vi "test Verify with Multi Scrubber.vi"(8 "error in":errorcluster, 11 "Test Case In":refnum<class "LUnit Extensions Tests.lvclass">) -> (0 "error out":errorcluster, 3 "Test Case Out":refnum<class "LUnit Extensions Tests.lvclass">)   [LabVIEW 2020, in "LUnit Extensions Tests.lvclass"]
uses:
  LUnit Extensions Tests.lvclass
  LUnit Extensions Tests.lvclass/LUnit Extensions Tests.ctl
  240f995d-3744-484a-8956-6f48e6079b93.vi
  Source/Approval Tests/Regex Scrubber/Regex Scrubber.lvclass
  Source/Approval Tests/Options/Options.lvclass
  C:/Users/SAS/Desktop/ApprovalTests.LabVIEW/Source/Approval Tests/Regex Scrubber/Regex Scrubber.lvclass
  C:/Users/SAS/Desktop/ApprovalTests.LabVIEW/Source/Approval Tests/Scrubber/Scrubber.lvclass
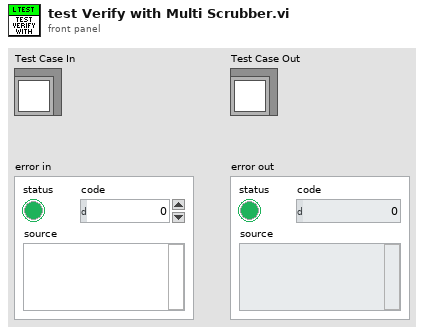
[diagram p1: front panel]
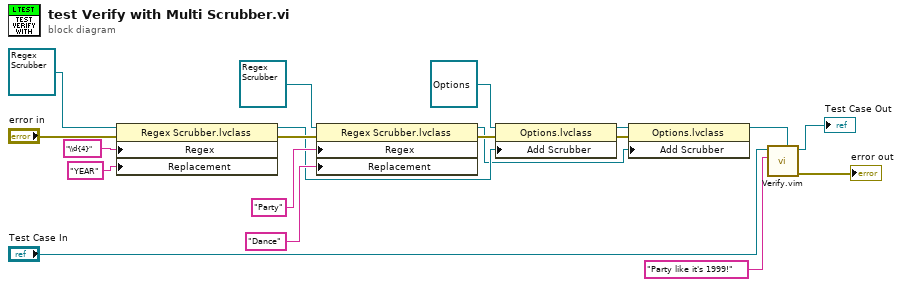
[diagram p0: block diagram]
diagram:
  n1 = property class="Regex Scrubber.lvclass"(reference=refnum<class "Regex Scrubber.lvclass"> refnum ("Approval Tests.lvlib:Regex Scrubber.lvclass"), error in="error in", "Regex"="\\d{4}", "Replacement"="YEAR") -> (reference out=w5:refnum<class "Regex Scrubber.lvclass">, error out=w18:errorcluster)
  n2 = property class="Regex Scrubber.lvclass"(reference=refnum<class "Regex Scrubber.lvclass"> refnum ("Approval Tests.lvlib:Regex Scrubber.lvclass"), error in=w18, "Regex"="Party", "Replacement"="Dance") -> (reference out=w2:refnum<class "Regex Scrubber.lvclass">, error out=w6:errorcluster)
  n3 = property class="Options.lvclass"(reference=refnum<class "Options.lvclass"> refnum ("Approval Tests.lvlib:Options.lvclass"), error in=w6, "Add Scrubber"=w5) -> (reference out=w4:refnum<class "Options.lvclass">, error out=w3:errorcluster)
  n4 = property class="Options.lvclass"(reference=w4, error in=w3, "Add Scrubber"=w2) -> (reference out=w1:refnum<class "Options.lvclass">)  [unwired: 1 out]
  n5 = call "Verify.vim"("Options"=w1, "Test Data"="Party like it's 1999!", "LUnit Test Case In"="Test Case In") -> ("error out"=→"error out":errorcluster, "LUnit Test Case Out"=→"Test Case Out":refnum<class "LUnit Extensions Tests.lvclass">)  [unwired: 7 in]
